vi "micro_Devices.vi"() -> ()   [LabVIEW 2021]
doc: "André Romero - 2023\nandretec@ifsc.usp.br\nIFSC - USP"
uses:
  Controller.ctl
  Thorlabs-Vector-Move/aptTec/Thorlabs-V2/Global Motors.vi
panel:
  out "Z ini":dbl
  out "Array Structures Ind":refnum<vi>[](array[refnum])
  in  "Tab Control":T1(tab)=enum."Cubes"
  in  "start-stop":bool
  in  "step size (mm)":dbl=10.0
  in  "Min   Z":bool
  in  "Max  Z":bool
  in  "Min":bool
  in  "Max":bool
  in  "Z (m/s)":dbl=50.0
  in  "XY (m/s)":dbl format="%#_5g"
  out "Motor Y":bool=TRUE
  out "Motor X":bool=TRUE
  out "Motor Z":bool=TRUE
  in  "Motor - Z":refnum<k7>(container)
  in  "Motor - Y":refnum<k7>(container)
  in  "Motor - X":refnum<k7>(container)
  out "current cube":i32
  out "current Layer":i32=1
  out "Total Progress (%)":u8(slide) caption="Layer Progress (%)" scale=0.0..25.0
  out "Layer Progress (%)":u8(slide)=100 scale=0.0..100.0
  in  "Line step size (mm)":dbl=1.0
  out "Lines Progress (%)":u8(slide)=42 scale=0.0..100.0
  in  "Stop Button":bool
  in  "Go Cubes":bool
  in  "Array of Structures":bool
  in  "Velocity (m/s)":dbl=50.0
  out "Layers":dbl=1.0
  in  "Delta Y (um)":dbl=50.0
  in  "Delta X (um)":dbl=50.0
  in  "Number of Lines":i32=2
  in  "Number of Columns":i32=5
  in  "Layer height (mm)":dbl=1.0
  in  "Height (mm)":dbl=1.0
  in  "Length (mm)":dbl=20.0
  in  "Width (mm)":dbl=20.0
  out "X ini":dbl
  out "Y ini":dbl
  in  "Initial position Z":bool=TRUE
  in  "Z offset (mm)":dbl=10.0
  in  "Z offset":bool
  in  "Motor - Z2":refnum<k7>(container)
  in  "N Loops":i32=5
  in  "Velocity (m/s)":dbl=50.0
  in  "Line step size (mm)":dbl=1.0
  in  "Layer height (mm)":dbl=1.0
  in  "Height (mm)":dbl=5.0
  in  "Length (mm)":dbl=20.0
  in  "Width (mm)":dbl=20.0
  in  "Go Lens":bool
  in  "Release":bool
  out "Numeric":i32
  out "error out":errorcluster
  out "Position Z":sgl
  out "Position Y":dbl
  out "Position X":dbl
  in  "Scale (um)":dbl
  out "XY Graph":cluster{dbl[], dbl[]}(graph)
  in  "Go Test":bool
  in  "Density points":i32
  in  "Velocity (m/s)":dbl=50.0
  in  "círculos":i32
  in  "layers":i32
  in  "scale  z (um)":dbl
  # "Velocity"
  # "Jog"
  # "mm"
  # "Z"
  # "Settings"
  # "Control"
  # "Settings"
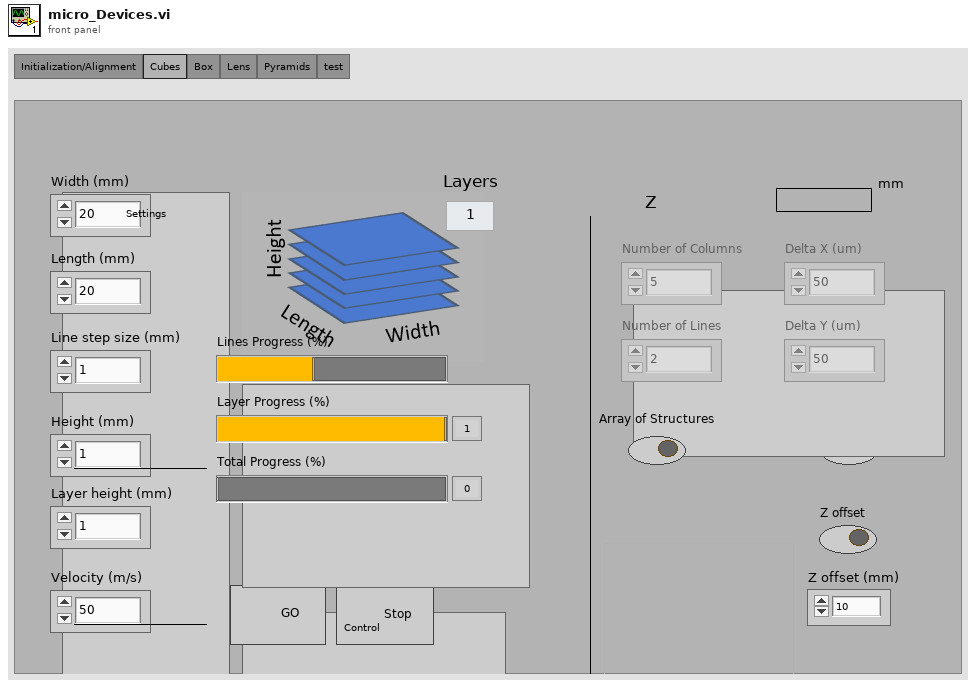
[diagram p1: front panel]
types:
  T1 = enum32{"Initialization/Alignment", "Cubes", "Box", "Lens", "Pyramids", "test"}
  T2 = typedef "Controller.ctl" = enum16{"Initialize", "Wait for Event", "Cubes", "Lens", "Box", "test tap"}
  T3 = typedef "eventvkey.ctl" = enum16{"ASCII", "Enter", "Return", "Shift", "Ctrl", "Alt", "Cmd", "Opt", "Caps", "NumLock", "Clear", "Break", "Up", "Down", "Left", "Right", "Insert", "Delete", "Home", "End", "PageUp", "PageDown", "Escape", "Help", "Pause", "ScrollLock", "F1", "F2", "F3", "F4", "F5", "F6", "F7", "F8", "F9", "F10", "F11", "F12", "F13", "F14", "F15", "F16", "F17", "F18", "F19", "F20", "F21", "F22", "F23", "F24", "Play", "VolumeUp", "VolumeDown", "Mute", "Two Byte Char"}
  T4 = enum8{"Enabled", "Disabled", "Disabled and Grayed Out"}
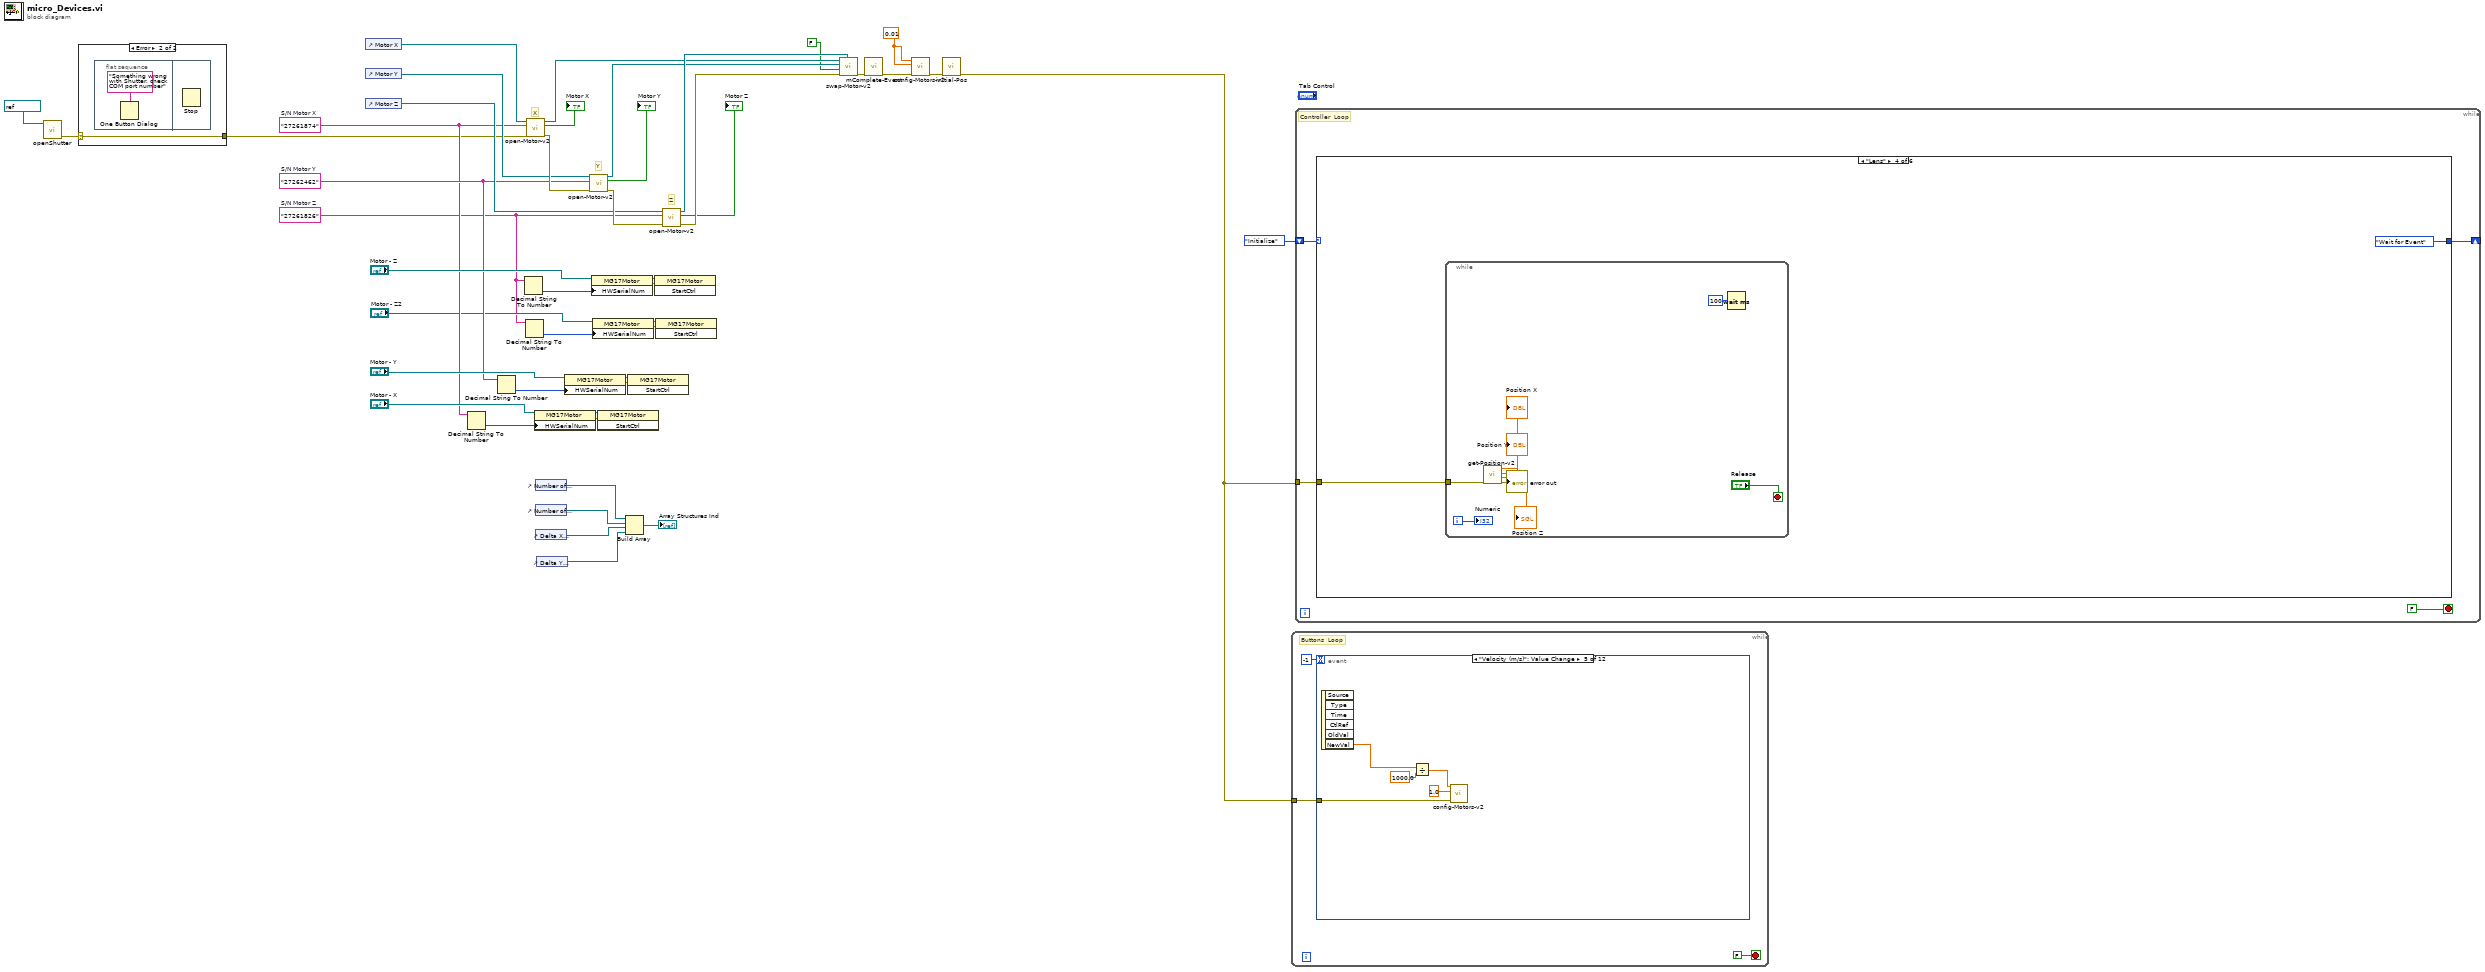
[diagram p0: block diagram]
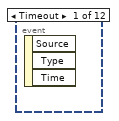
[diagram p3: hidden frame]
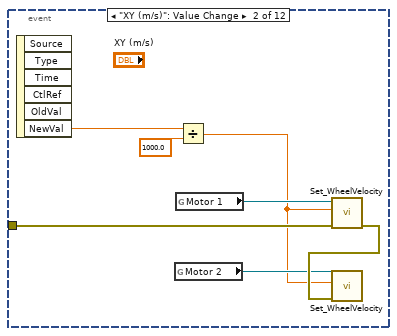
[diagram p4: hidden frame]
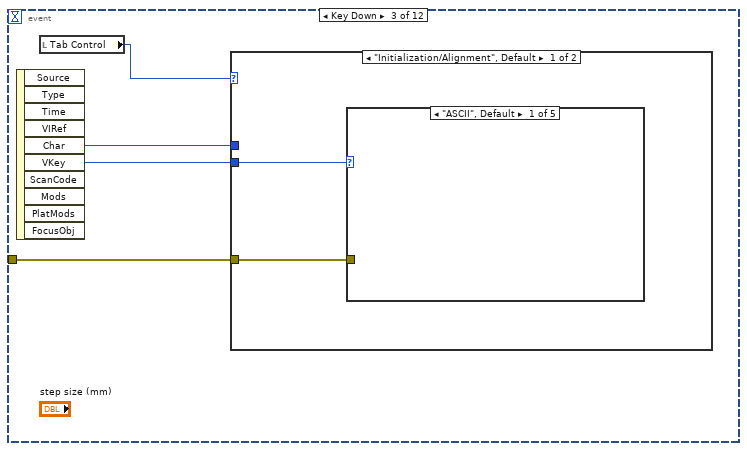
[diagram p5: hidden frame]
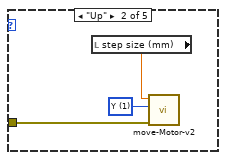
[diagram p6: hidden frame]
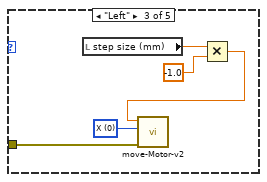
[diagram p7: hidden frame]
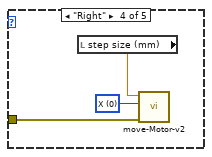
[diagram p8: hidden frame]
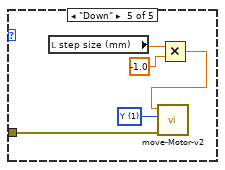
[diagram p9: hidden frame]
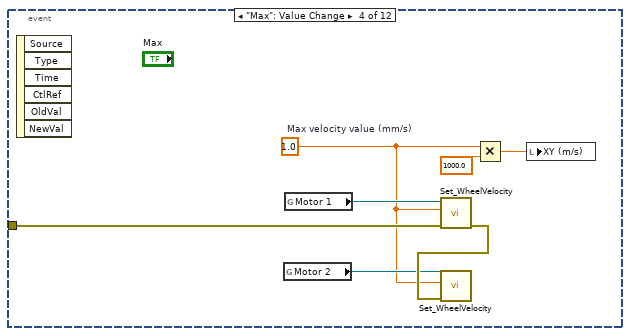
[diagram p11: hidden frame]
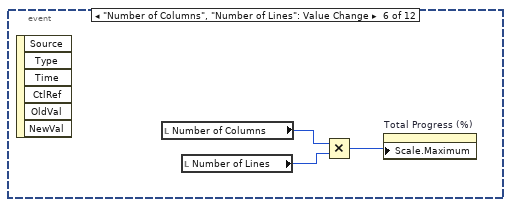
[diagram p12: hidden frame]
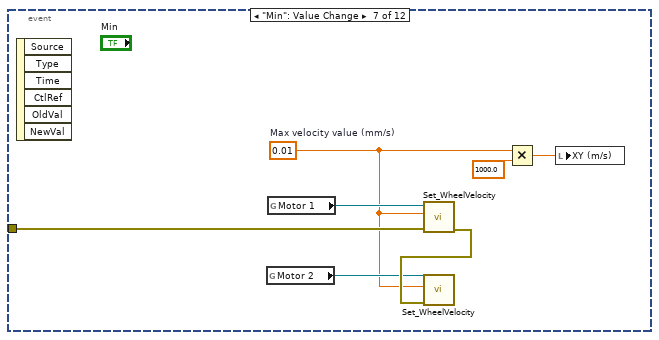
[diagram p13: hidden frame]
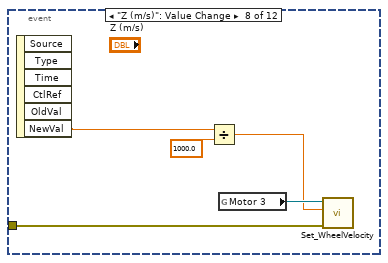
[diagram p14: hidden frame]
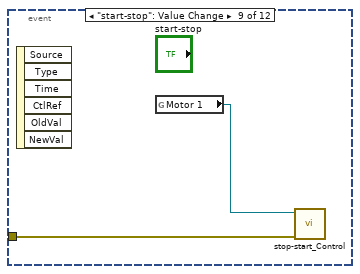
[diagram p15: hidden frame]
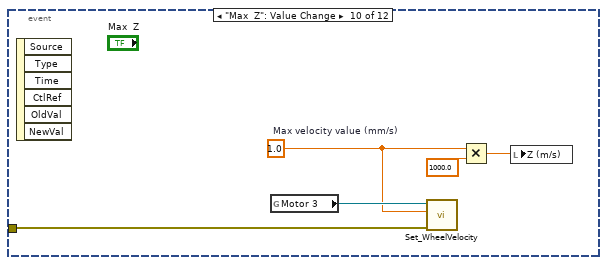
[diagram p16: hidden frame]
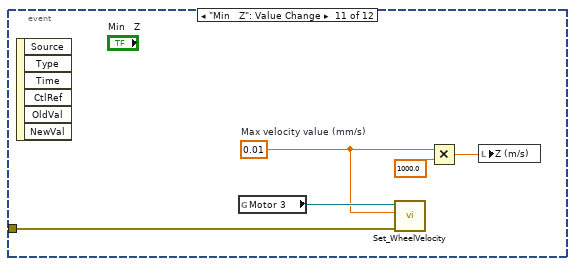
[diagram p17: hidden frame]
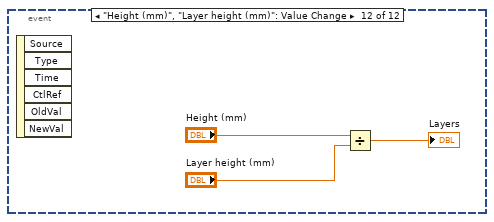
[diagram p18: hidden frame]
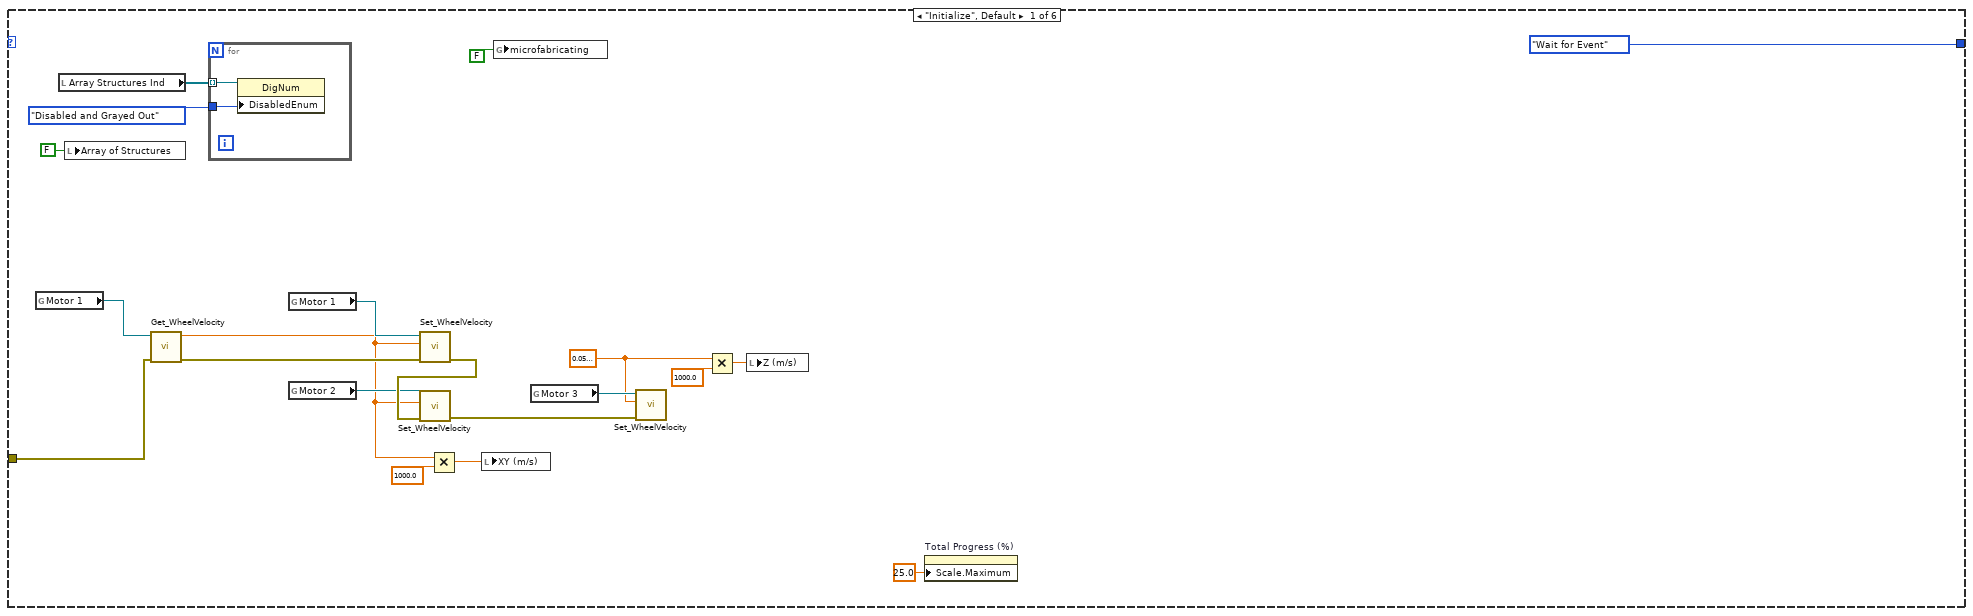
[diagram p19: hidden frame]
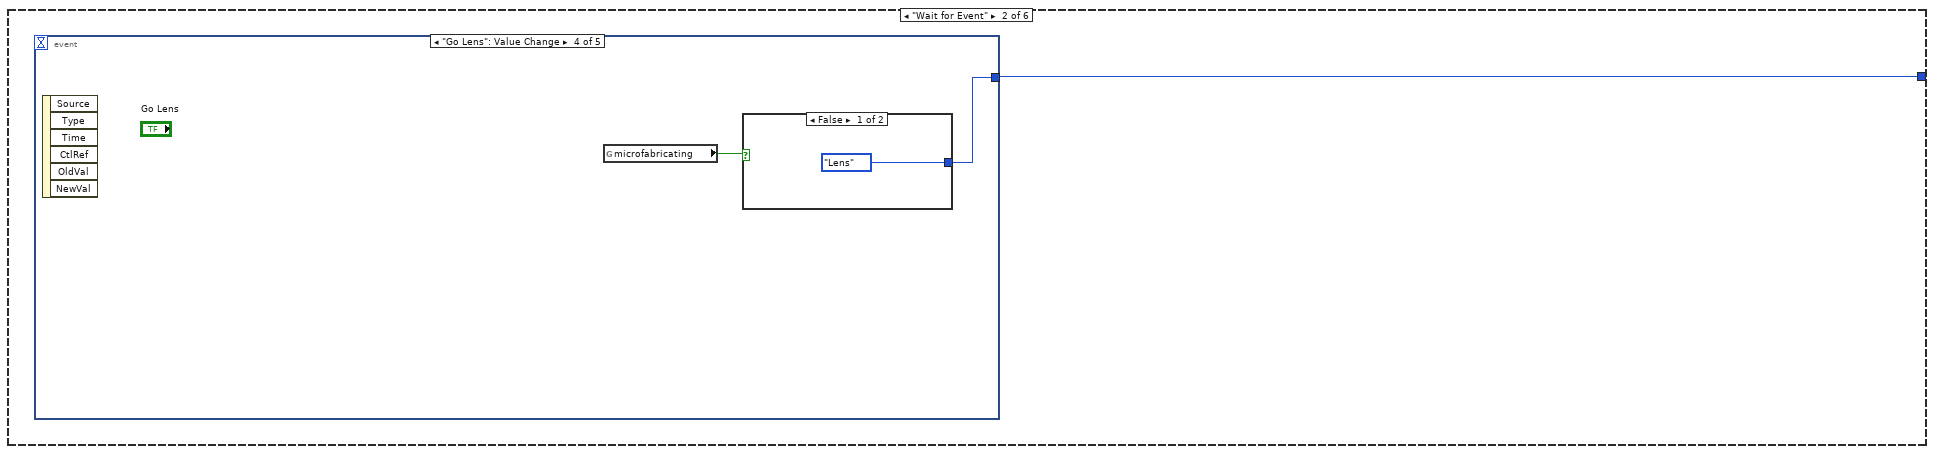
[diagram p20: hidden frame]
diagram:
  w29 = 0.01 ("Acc")
  w16 = "27262462"  # S/N Motor Y
  w15 = "27261874"  # S/N Motor X
  w1 = "27261826"  # S/N Motor Z
  # "X"
  # "Y"
  # "Z"
  n1 = call "openShutter.vi"("VISA Refnum in"=refnum<visa-resource-name> "COM3") -> ("error out"=w7:errorcluster)  [unwired: 9 in, 1 out]
  n2 = case shown="Error" w7 {
    selector: w7 -> [w47 w48]
    tunnel: [w47 w48] -> w6
    frame No Error {
    }
    frame Error {
      n3 = flat-sequence {
        frame #0 {
          n4 = One Button Dialog(message="Something wrong with Shutter, check COM port number") -> ()  [unwired: 1 in, 1 out]
        }
        frame #1 {
          n5 = Stop() -> ()  [unwired: 1 in]
        }
      }
    }
  }
  n6 = control-ref of="Motor X"() -> (w43:refnum<vi>)
  n7 = control-ref of="Motor Y"() -> (w42:refnum<vi>)
  n8 = control-ref of="Motor Z"() -> (w38:refnum<vi>)
  n9 = Decimal String To Number(string=w15) -> (number=w17:i32)  [unwired: 2 in, 1 out]
  n10 = Decimal String To Number(string=w16) -> (number=w21:i32)  [unwired: 2 in, 1 out]
  n11 = Decimal String To Number(string=w1) -> (number=w25:i32)  [unwired: 2 in, 1 out]
  n12 = Decimal String To Number(string=w1) -> (number=w2:i32)  [unwired: 2 in, 1 out]
  n13 = call "open-Motor-v2.vi"("Error In"=w6, "S/N Motor"=w15, "ref Boolean in"=w43) -> ("Error Out"=w46:errorcluster, "Motor Status"=→"Motor X":bool, "Refnum out"=w11:refnum<k7>)  [unwired: 6 in]
  n14 = property class="MG17Motor"(reference="Motor - X", "HWSerialNum"=w17) -> (reference out=w18:refnum<k7>, error out=w19:errorcluster)  [unwired: 1 in]
  n15 = control-ref of="Number of Lines"() -> (w34:refnum<vi>)
  n16 = control-ref of="Number of Columns"() -> (w33:refnum<vi>)
  n17 = control-ref of="Delta X (um)"() -> (w32:refnum<vi>)
  n18 = control-ref of="Delta Y (um)"() -> (w31:refnum<vi>)
  n19 = property class="MG17Motor"(reference="Motor - Y", "HWSerialNum"=w21) -> (reference out=w22:refnum<k7>, error out=w23:errorcluster)  [unwired: 1 in]
  n20 = call "open-Motor-v2.vi"("Error In"=w46, "S/N Motor"=w16, "ref Boolean in"=w42) -> ("Error Out"=w40:errorcluster, "Motor Status"=→"Motor Y":bool, "Refnum out"=w10:refnum<k7>)  [unwired: 6 in]
  n21 = property class="MG17Motor"(reference="Motor - Z", "HWSerialNum"=w25) -> (reference out=w26:refnum<k7>, error out=w27:errorcluster)  [unwired: 1 in]
  n22 = property class="MG17Motor"(reference="Motor - Z2", "HWSerialNum"=w2) -> (reference out=w3:refnum<k7>, error out=w4:errorcluster)  [unwired: 1 in]
  n23 = invoke class="MG17Motor" method="StartCtrl"(reference=w18, error in=w19) -> ()  [unwired: 1 in, 3 out]
  n24 = Build Array(w34, w33, w32, w31) -> (→"Array Structures Ind":refnum<vi>[])
  n25 = invoke class="MG17Motor" method="StartCtrl"(reference=w22, error in=w23) -> ()  [unwired: 1 in, 3 out]
  n26 = invoke class="MG17Motor" method="StartCtrl"(reference=w26, error in=w27) -> ()  [unwired: 1 in, 3 out]
  n27 = invoke class="MG17Motor" method="StartCtrl"(reference=w3, error in=w4) -> ()  [unwired: 1 in, 3 out]
  n28 = call "open-Motor-v2.vi"("Error In"=w40, "S/N Motor"=w1, "ref Boolean in"=w38) -> ("Error Out"=w39:errorcluster, "Motor Status"=→"Motor Z":bool, "Refnum out"=w36:refnum<k7>)  [unwired: 6 in]
  n29 = call "swap-Motor-v2.vi"("Refnum in M3"=w36, "error in (no error)"=w39, "Swap motor"=FALSE, "Refnum in M2"=w10, "Refnum in M1"=w11) -> ("error out"=w14:errorcluster)  [unwired: 6 in]
  n30 = call "mComplete-Event.vi"("Error In"=w14) -> ("Error Out"=w13:errorcluster)  [unwired: 10 in]
  n31 = call "config-Motors-v2.vi"("error in"=w13, "Acc"=w29, "Velocity"=w29) -> ("error out"=w41:errorcluster)  [unwired: 8 in]
  n32 = call "initial-Pos.vi"("error in (no error)"=w41) -> ("error out"=w12:errorcluster)  [unwired: 10 in]
  n33 = while {
    tunnel: w12 -> [w51]
    stop <- FALSE stop-if-true
    # "Buttons  Loop"
    n34 = event shown="[4] \"Velocity (m/s)\": Value Change" {
      selector: _ -> [_ _ _ _ _ _ _ _ _ _ _ _]
      dyn-events: _ -> [_ _ _ _ _ _ _ _ _ _ _ _]
      timeout: -1 -> [_ _ _ _ _ _ _ _ _ _ _ _]
      tunnel: w51 -> [_ w58 w60 w85 w89 _ w100 w104 w110 w111 w116 _]
      event Timeout {
        n35 = event-data() -> ()  [unwired: 1 in, 3 out]
      }
      event "XY (m/s)": Value Change {
        n36 = event-data() -> ("NewVal"=w55:dbl)  [unwired: 1 in, 5 out]
        n37 = global read "Global Motors.vi" "Motor 2"() -> (w56:refnum<k7>)
        n38 = global read "Global Motors.vi" "Motor 1"() -> (w59:refnum<k7>)
        n39 = Divide(x=w55, y=1000.0) -> (x/y=w54:dbl)
        n40 = call "Set_WheelVelocity.vi"("error in"=w58, "fWheelVel"=w54, "MG17Motor in"=w59) -> ("error out"=w57:errorcluster)  [unwired: 8 in]
        n41 = call "Set_WheelVelocity.vi"("error in"=w57, "fWheelVel"=w54, "MG17Motor in"=w56) -> ()  [unwired: 8 in, 1 out]
      }
      event Key Down {
        n42 = event-data() -> ("Char"=w62:i16, "VKey"=w61:T3)  [unwired: 1 in, 8 out]
        n43 = local read "Tab Control"() -> (w63:T1)
        n44 = case shown="\"Initialization/Alignment\", Default" w63 {
          tunnel: w62 -> [_ _]
          tunnel: w61 -> [w65 _]
          tunnel: w60 -> [w64 _]
          frame "Initialization/Alignment", Default {
            n45 = case shown="\"ASCII\", Default" w65 {
              tunnel: w64 -> [_ w68 w73 w76 w80]
              frame "ASCII", Default {
              }
              frame "Up" {
                w67 = u16 1 items=["X", "Y", "Z"] ("Axis")
                n46 = local read "step size (mm)"() -> (w66:dbl)
                n47 = call "move-Motor-v2.vi"("error in"=w68, "Axis"=w67, "Distance (um)"=w66) -> ()  [unwired: 8 in, 1 out]
              }
              frame "Left" {
                w72 = u16 0 items=["X", "Y", "Z"] ("Axis")
                n48 = local read "step size (mm)"() -> (w71:dbl)
                n49 = Multiply(x=w71, y=-1.0) -> (x*y=w69:dbl)
                n50 = call "move-Motor-v2.vi"("error in"=w73, "Axis"=w72, "Distance (um)"=w69) -> ()  [unwired: 8 in, 1 out]
              }
              frame "Right" {
                w75 = u16 0 items=["X", "Y", "Z"] ("Axis")
                n51 = local read "step size (mm)"() -> (w74:dbl)
                n52 = call "move-Motor-v2.vi"("error in"=w76, "Axis"=w75, "Distance (um)"=w74) -> ()  [unwired: 8 in, 1 out]
              }
              frame "Down" {
                w81 = u16 1 items=["X", "Y", "Z"] ("Axis")
                n53 = local read "step size (mm)"() -> (w79:dbl)
                n54 = Multiply(x=w79, y=-1.0) -> (x*y=w77:dbl)
                n55 = call "move-Motor-v2.vi"("error in"=w80, "Axis"=w81, "Distance (um)"=w77) -> ()  [unwired: 8 in, 1 out]
              }
            }
          }
          frame "Cubes" {
          }
        }
      }
      event "Max": Value Change {
        w83 = 1.0  # Max velocity value (mm/s)
        n56 = event-data() -> ()  [unwired: 1 in, 6 out]
        n57 = global read "Global Motors.vi" "Motor 2"() -> (w86:refnum<k7>)
        n58 = global read "Global Motors.vi" "Motor 1"() -> (w88:refnum<k7>)
        n59 = call "Set_WheelVelocity.vi"("error in"=w85, "fWheelVel"=w83, "MG17Motor in"=w88) -> ("error out"=w87:errorcluster)  [unwired: 8 in]
        n60 = call "Set_WheelVelocity.vi"("error in"=w87, "fWheelVel"=w83, "MG17Motor in"=w86) -> ()  [unwired: 8 in, 1 out]
        n61 = Multiply(x=w83, y=1000.0) -> (x*y=w82:dbl)
        n62 = local write "XY (m/s)"(w82) -> ()
      }
      event "Velocity (m/s)": Value Change {
        n63 = event-data() -> ("NewVal"=w93:dbl)  [unwired: 1 in, 5 out]
        n64 = Divide(x=w93, y=1000.0) -> (x/y=w91:dbl)
        n65 = call "config-Motors-v2.vi"("error in"=w89, "Acc"=1.0, "Velocity"=w91) -> ()  [unwired: 8 in, 1 out]
      }
      event "Number of Columns", "Number of Lines": Value Change {
        n66 = event-data() -> ()  [unwired: 1 in, 6 out]
        n67 = local read "Number of Columns"() -> (w95:i32)
        n68 = local read "Number of Lines"() -> (w96:i32)
        n69 = Multiply(x=w95, y=w96) -> (x*y=w94:i32)
        n70 = property on="Total Progress (%)" class="Slide (strict)"("Scale.Maximum"=w94) -> ()  [unwired: 2 in, 2 out]
      }
      event "Min": Value Change {
        w98 = 0.01  # Max velocity value (mm/s)
        n71 = event-data() -> ()  [unwired: 1 in, 6 out]
        n72 = global read "Global Motors.vi" "Motor 2"() -> (w101:refnum<k7>)
        n73 = global read "Global Motors.vi" "Motor 1"() -> (w103:refnum<k7>)
        n74 = call "Set_WheelVelocity.vi"("error in"=w100, "fWheelVel"=w98, "MG17Motor in"=w103) -> ("error out"=w102:errorcluster)  [unwired: 8 in]
        n75 = call "Set_WheelVelocity.vi"("error in"=w102, "fWheelVel"=w98, "MG17Motor in"=w101) -> ()  [unwired: 8 in, 1 out]
        n76 = Multiply(x=w98, y=1000.0) -> (x*y=w97:dbl)
        n77 = local write "XY (m/s)"(w97) -> ()
      }
      event "Z (m/s)": Value Change {
        n78 = event-data() -> ("NewVal"=w107:dbl)  [unwired: 1 in, 5 out]
        n79 = Divide(x=w107, y=1000.0) -> (x/y=w105:dbl)
        n80 = global read "Global Motors.vi" "Motor 3"() -> (w106:refnum<k7>)
        n81 = call "Set_WheelVelocity.vi"("error in"=w104, "fWheelVel"=w105, "MG17Motor in"=w106) -> ()  [unwired: 8 in, 1 out]
      }
      event "start-stop": Value Change {
        n82 = event-data() -> ()  [unwired: 1 in, 6 out]
        n83 = global read "Global Motors.vi" "Motor 1"() -> (w109:refnum<k7>)
        n84 = call "stop-start_Control.vi"("error in (no error)"=w110, "Automation Refnum in"=w109) -> ()  [unwired: 8 in, 2 out]
      }
      event "Max  Z": Value Change {
        w113 = 1.0  # Max velocity value (mm/s)
        n85 = event-data() -> ()  [unwired: 1 in, 6 out]
        n86 = global read "Global Motors.vi" "Motor 3"() -> (w115:refnum<k7>)
        n87 = call "Set_WheelVelocity.vi"("error in"=w111, "fWheelVel"=w113, "MG17Motor in"=w115) -> ()  [unwired: 8 in, 1 out]
        n88 = Multiply(x=w113, y=1000.0) -> (x*y=w112:dbl)
        n89 = local write "Z (m/s)"(w112) -> ()
      }
      event "Min   Z": Value Change {
        w118 = 0.01  # Max velocity value (mm/s)
        n90 = event-data() -> ()  [unwired: 1 in, 6 out]
        n91 = global read "Global Motors.vi" "Motor 3"() -> (w120:refnum<k7>)
        n92 = call "Set_WheelVelocity.vi"("error in"=w116, "fWheelVel"=w118, "MG17Motor in"=w120) -> ()  [unwired: 8 in, 1 out]
        n93 = Multiply(x=w118, y=1000.0) -> (x*y=w117:dbl)
        n94 = local write "Z (m/s)"(w117) -> ()
      }
      event "Height (mm)", "Layer height (mm)": Value Change {
        n95 = event-data() -> ()  [unwired: 1 in, 6 out]
        n96 = Divide(x="Height (mm)", y="Layer height (mm)") -> (x/y=→"Layers":dbl)
      }
    }
  }
  n97 = while {
    shift-right: [w125] -> _
    shift-left: Controller."Initialize" -> [w126]
    tunnel: w12 -> [w124]
    stop <- FALSE stop-if-true
    # "Controller  Loop"
    n98 = case shown="\"Lens\"" w126 {
      tunnel: [Controller."Wait for Event" w150 Controller."Wait for Event" Controller."Wait for Event" Controller."Wait for Event" w362] -> w125
      tunnel: w124 -> [w129 _ w191 w326 w338 w355]
      frame "Initialize", Default {
        w133 = sgl 0.05 ("fWheelVel")
        n99 = global read "Global Motors.vi" "Motor 1"() -> (w143:refnum<k7>)
        n100 = local read "Array Structures Ind"() -> (w145:refnum<vi>[])
        n101 = local write "Array of Structures"(FALSE ("Array of Structures")) -> ()
        n102 = call "Get_WheelVelocity.vi"("error in"=w129, "MG17Motor in"=w143) -> ("error out"=w139:errorcluster, "pfWheelVel"=w138:sgl)  [unwired: 8 in]
        n103 = for {
          tunnel: T4."Disabled and Grayed Out" ("Disabled") -> [w149]
          tunnel: w145 -> [w148] mode=indexing
          n104 = property class="DigNum"(reference=w148, "DisabledEnum"=w149) -> ()  [unwired: 1 in, 2 out]
        }
        n105 = global read "Global Motors.vi" "Motor 1"() -> (w142:refnum<k7>)
        n106 = global read "Global Motors.vi" "Motor 2"() -> (w140:refnum<k7>)
        n107 = call "Set_WheelVelocity.vi"("error in"=w139, "fWheelVel"=w138, "MG17Motor in"=w142) -> ("error out"=w141:errorcluster)  [unwired: 8 in]
        n108 = call "Set_WheelVelocity.vi"("error in"=w141, "fWheelVel"=w138, "MG17Motor in"=w140) -> ("error out"=w135:errorcluster)  [unwired: 8 in]
        n109 = Multiply(x=w138, y=sgl 1000.0) -> (x*y=w137:sgl)
        n110 = local write "XY (m/s)"(w137) -> ()
        n111 = global write "Global micro_Devices.vi" "microfabricating"(FALSE ("microfabricating")) -> ()
        n112 = global read "Global Motors.vi" "Motor 3"() -> (w134:refnum<k7>)
        n113 = call "Set_WheelVelocity.vi"("error in"=w135, "fWheelVel"=w133, "MG17Motor in"=w134) -> ()  [unwired: 8 in, 1 out]
        n114 = Multiply(x=w133, y=sgl 1000.0) -> (x*y=w132:sgl)
        n115 = local write "Z (m/s)"(w132) -> ()
        n116 = property on="Total Progress (%)" class="Slide (strict)"("Scale.Maximum"=25.0 ("Scale.Range:Maximum")) -> ()  [unwired: 2 in, 2 out]
      }
      frame "Wait for Event" {
        n117 = event shown="[3] \"Go Lens\": Value Change" {
          selector: _ -> [_ _ _ _ _]
          dyn-events: _ -> [_ _ _ _ _]
          timeout: _ -> [_ _ _ _ _]
          tunnel: [Controller."Wait for Event" Controller."Wait for Event" w160 w164 w168] -> w150
          event Timeout {
            n118 = event-data() -> ()  [unwired: 1 in, 3 out]
          }
          event "Array of Structures": Value Change {
            n119 = event-data() -> ("NewVal"=w153:bool)  [unwired: 1 in, 5 out]
            n120 = case shown="False" w153 {
              tunnel: [T4."Disabled and Grayed Out" ("Disabled") T4."Enabled" ("Disabled")] -> w154
              frame False {
              }
              frame True {
              }
            }
            n121 = local read "Array Structures Ind"() -> (w155:refnum<vi>[])
            n122 = for {
              tunnel: w154 -> [w157]
              tunnel: w155 -> [w156] mode=indexing
              n123 = property class="DigNum"(reference=w156, "DisabledEnum"=w157) -> ()  [unwired: 1 in, 2 out]
            }
          }
          event "Go Cubes": Value Change {
            n124 = event-data() -> ()  [unwired: 1 in, 6 out]
            n125 = global read "Global micro_Devices.vi" "microfabricating"() -> (w161:bool)
            n126 = case shown="False" w161 {
              tunnel: [Controller."Cubes" Controller."Wait for Event"] -> w160
              frame False {
              }
              frame True {
              }
            }
          }
          event "Go Lens": Value Change {
            n127 = event-data() -> ()  [unwired: 1 in, 6 out]
            n128 = global read "Global micro_Devices.vi" "microfabricating"() -> (w165:bool)
            n129 = case shown="False" w165 {
              tunnel: [Controller."Lens" Controller."Wait for Event"] -> w164
              frame False {
              }
              frame True {
              }
            }
          }
          event "Go Test": Value Change {
            n130 = event-data() -> ()  [unwired: 1 in, 6 out]
            n131 = global read "Global micro_Devices.vi" "microfabricating"() -> (w169:bool)
            n132 = case shown="True" w169 {
              tunnel: [Controller."test tap" Controller."Wait for Event"] -> w168
              frame False {
              }
              frame True {
              }
            }
          }
        }
      }
      frame "Cubes" {
        w178 = u16 1 items=["X", "Y", "Z"] ("Axis")
        w177 = 0.0 ("Distance (um)")
        w180 = u16 0 items=["X", "Y", "Z"] ("Axis")
        # "Initial Settings"
        # "Backlash"
        n133 = global write "Global micro_Devices.vi" "Current Cube"(1 ("Current Cube")) -> ()
        n134 = global write "Global micro_Devices.vi" "microfabricating"(FALSE ("microfabricating")) -> ()
        n135 = Divide(x="Velocity (m/s)", y=1000.0) -> (x/y=w182:dbl)
        n136 = call "config-Motors-v2.vi"("error in"=w191, "Acc"=1.0, "Velocity"=w182) -> ("error out"=w176:errorcluster)  [unwired: 8 in]
        n137 = call "move-Motor-v2.vi"("error in"=w176, "Axis"=w180, "Distance (um)"=w177) -> ("error out"=w179:errorcluster)  [unwired: 8 in]
        n138 = call "move-Motor-v2.vi"("error in"=w179, "Axis"=w178, "Distance (um)"=w177) -> ("error out"=w175:errorcluster)  [unwired: 8 in]
        n139 = Multiply(x=1.0, y="Width (mm)") -> (x*y=w173:dbl)
        n140 = local read "Array of Structures"() -> (w186:bool)
        n141 = call "initial-Pos-XY.vi"("error in (no error)"=w175) -> ("error out"=w188:errorcluster, "Y position"=w184:dbl, "X position"=w185:dbl)  [unwired: 8 in]
        n142 = Divide(x="Length (mm)", y="Line step size (mm)") -> (x/y=w193:dbl)
        n143 = call "initial-Pos-Z.vi"("error in (no error)"=w188) -> ("error out"=w187:errorcluster, "Z position"=w183:dbl)  [unwired: 9 in]
        n144 = case shown="True" w186 {
          tunnel: w173 -> [w203 w238]
          tunnel: w193 -> [w202 w239]
          tunnel: "Line step size (mm)" -> [w201 w237]
          tunnel: w187 -> [w200 w236]
          tunnel: w185 -> [_ w235]
          tunnel: w184 -> [_ w234]
          tunnel: w183 -> [_ w233]
          frame False {
            n145 = while {
              tunnel: w203 -> [w225]
              tunnel: w202 -> [w224]
              tunnel: w201 -> [w223]
              tunnel: w200 -> [w221]
              tunnel: [w214] -> w199
              i -> [w217]
              stop <- w216 stop-if-true
              n146 = call "toggleShutter.vi"("Error In"=w221) -> ("error out"=w220:errorcluster)  [unwired: 9 in]
              n147 = Increment(x=w217) -> (x+1=w212:i32)
              "current Layer" <- w212
              n148 = local read "Layer height (mm)"() -> (w208:dbl)
              n149 = local read "Height (mm)"() -> (w207:dbl)
              n150 = control-ref of="Lines Progress (%)"() -> (w222:refnum<vi>)
              n151 = Multiply(x=100.0, y=w212) -> (x*y=w211:dbl)
              n152 = call "make-Lines.vi"("Shutter off between lines"=TRUE, "Slide in"=w222, "error in"=w220, "d (um)"=w223, "L (um)"=w225, "N Lines"=w224) -> ("error out"=w219:errorcluster)  [unwired: 4 in, 1 out]
              n153 = call "toggleShutter.vi"("Error In"=w219) -> ("error out"=w218:errorcluster)  [unwired: 9 in]
              n154 = local read "Layers"() -> (w210:dbl)
              n155 = Equal?(x=w207, y=w208) -> (x = y?=w206:bool)
              n156 = Divide(x=w211, y=w210) -> (x/y=→"Layer Progress (%)":dbl)
              n157 = case shown="False" w206 {
                tunnel: w218 -> [w228 w230]
                tunnel: [w227 w230] -> w215
                tunnel: w208 -> [w226 _]
                frame False {
                  w229 = u16 2 items=["X", "Y", "Z"] ("Axis")
                  n158 = call "move-Motor-v2.vi"("error in"=w228, "Axis"=w229, "Distance (um)"=w226) -> ("error out"=w227:errorcluster)  [unwired: 8 in]
                }
                frame True {
                }
              }
              n159 = Equal?(x=w210, y=w212) -> (x = y?=w216:bool)
              n160 = call "moveXYToInitialPos.vi"("error in"=w215) -> ("error out"=w214:errorcluster)  [unwired: 10 in]
            }
            n161 = case shown="True" "Initial position Z" {
              tunnel: w199 -> [_ w204]
              frame False {
              }
              frame True {
                n162 = call "moveZToInitialPos.vi"("error in"=w204) -> ()  [unwired: 10 in, 1 out]
              }
            }
          }
          frame True {
            n163 = while {
              tunnel: w239 -> [w260]
              tunnel: w238 -> [w259]
              tunnel: w237 -> [w258]
              tunnel: w236 -> [w257]
              tunnel: [w241] -> w231
              i -> [w254]
              stop <- w253 stop-if-true
              w252 = u16 1 items=["X", "Y", "Z"] ("Axis")
              n164 = while {
                tunnel: w260 -> [w289]
                tunnel: w259 -> [w288]
                tunnel: w258 -> [w287]
                tunnel: w257 -> [w286]
                tunnel: [w269] -> w242
                i -> [w279]
                stop <- w277 stop-if-true
                w284 = u16 0 items=["X", "Y", "Z"] ("Axis")
                n165 = global read "Global micro_Devices.vi" "Current Cube"() -> (w261:i32)
                "current cube" <- w261
                "Total Progress (%)" <- w261
                n166 = while {
                  tunnel: w289 -> [w317]
                  tunnel: w288 -> [w316]
                  tunnel: w287 -> [w315]
                  tunnel: w286 -> [w314]
                  tunnel: [w312] -> w285
                  i -> [w307]
                  stop <- w306 stop-if-true
                  n167 = control-ref of="Lines Progress (%)"() -> (w305:refnum<vi>)
                  n168 = call "toggleShutter.vi"("Error In"=w314) -> ("error out"=w313:errorcluster)  [unwired: 9 in]
                  n169 = Increment(x=w307) -> (x+1=w304:i32)
                  n170 = local read "Layer height (mm)"() -> (w302:dbl)
                  n171 = local read "Height (mm)"() -> (w301:dbl)
                  n172 = call "make-Lines.vi"("Shutter off between lines"=TRUE, "Slide in"=w305, "error in"=w313, "d (um)"=w315, "L (um)"=w316, "N Lines"=w317) -> ("error out"=w320:errorcluster)  [unwired: 4 in, 1 out]
                  n173 = Multiply(x=100.0, y=w304) -> (x*y=w309:dbl)
                  n174 = call "toggleShutter.vi"("Error In"=w320) -> ("error out"=w319:errorcluster)  [unwired: 9 in]
                  n175 = local write "current Layer"(w304) -> ()
                  n176 = Equal?(x=w302, y=w301) -> (x = y?=w303:bool)
                  n177 = local read "Layers"() -> (w310:dbl)
                  n178 = case shown="False" w303 {
                    tunnel: w319 -> [w323 w325]
                    tunnel: [w322 w325] -> w318
                    tunnel: w302 -> [w321 _]
                    frame False {
                      w324 = u16 2 items=["X", "Y", "Z"] ("Axis")
                      n179 = call "move-Motor-v2.vi"("error in"=w323, "Axis"=w324, "Distance (um)"=w321) -> ("error out"=w322:errorcluster)  [unwired: 8 in]
                    }
                    frame True {
                    }
                  }
                  n180 = Divide(x=w309, y=w310) -> (x/y=w308:dbl)
                  n181 = local write "Layer Progress (%)"(w308) -> ()
                  n182 = Greater Or Equal?(x=w310, y=w304) -> (x >= y?=w306:bool)
                  n183 = call "moveXYToInitialPos.vi"("error in"=w318) -> ("error out"=w312:errorcluster)  [unwired: 10 in]
                }
                n184 = Increment(x=w261) -> (x+1=w274:i32)
                n185 = global write "Global micro_Devices.vi" "Current Cube"(w274) -> ()
                n186 = local read "Width (mm)"() -> (w282:dbl)
                n187 = Multiply(x="Delta X (um)", y=1.0) -> (x*y=w273:dbl)
                n188 = Add(x=w282, y=w273) -> (x+y=w280:dbl)
                n189 = call "moveZToInitialPos.vi"("error in"=w285) -> ("error out"=w283:errorcluster)  [unwired: 10 in]
                n190 = global read "Global micro_Devices.vi" "Current Cube"() -> (w266:i32)
                n191 = local read "Z ini"() -> (w265:dbl)
                n192 = call "move-Motor-v2.vi"("error in"=w283, "Axis"=w284, "Distance (um)"=w280) -> ("error out"=w276:errorcluster)  [unwired: 8 in]
                n193 = call "initial-Pos-XY.vi"("error in (no error)"=w276) -> ("error out"=w270:errorcluster)  [unwired: 8 in, 2 out]
                n194 = Increment(x=w279) -> (x+1=w278:i32)
                n195 = Decrement(x=w266) -> (x-1=w267:i32)
                n196 = Multiply(x=w267, y="Z offset (mm)") -> (x*y=w264:dbl)
                n197 = Add(x=w264, y=w265) -> (x+y=w262:dbl)
                n198 = Equal?(x="Number of Columns", y=w278) -> (x = y?=w277:bool)
                n199 = Not Equal To 0?(x=w264) -> (x != 0?=w263:bool)
                n200 = case shown="True" "Z offset" {
                  tunnel: w270 -> [w290 w294]
                  tunnel: [w290 w293] -> w269
                  tunnel: w263 -> [_ w292]
                  tunnel: w262 -> [_ w291]
                  frame False {
                  }
                  frame True {
                    n201 = case shown="True" w292 {
                      tunnel: w294 -> [w295 w298]
                      tunnel: [w295 w297] -> w293
                      tunnel: w291 -> [_ w296]
                      frame False {
                      }
                      frame True {
                        w299 = u16 2 items=["X", "Y", "Z"] ("Axis")
                        n202 = call "move-Motor-v2.vi"("error in"=w298, "Axis"=w299, "Distance (um)"=w296) -> ("error out"=w297:errorcluster)  [unwired: 8 in]
                      }
                    }
                  }
                }
              }
              n203 = Increment(x=w254) -> (x+1=w248:i32)
              n204 = local read "X ini"() -> (w244:dbl)
              n205 = local read "Length (mm)"() -> (w255:dbl)
              n206 = Subtract(x=w244, y=0.02 ("x")) -> (x-y=w247:dbl)
              n207 = call "goToabsX.vi"("error in"=w242, "X position"=w247) -> ("error out"=w245:errorcluster)  [unwired: 9 in]
              n208 = Add(x="Delta Y (um)", y=w255) -> (x+y=w251:dbl)
              n209 = Equal?(x="Number of Lines", y=w248) -> (x = y?=w253:bool)
              n210 = call "goToabsX.vi"("error in"=w245, "X position"=w244) -> ("error out"=w243:errorcluster)  [unwired: 9 in]
              n211 = call "move-Motor-v2.vi"("error in"=w243, "Axis"=w252, "Distance (um)"=w251) -> ("error out"=w250:errorcluster)  [unwired: 8 in]
              n212 = call "initial-Pos-XY.vi"("error in (no error)"=w250) -> ("error out"=w241:errorcluster)  [unwired: 8 in, 2 out]
            }
            n213 = local read "Initial position Z"() -> (w232:bool)
            n214 = case shown="True" w232 {
              tunnel: w231 -> [_ w240]
              frame False {
              }
              frame True {
                n215 = call "moveZToInitialPos.vi"("error in"=w240) -> ()  [unwired: 10 in, 1 out]
              }
            }
            "X ini" <- w235
            "Y ini" <- w234
            "Z ini" <- w233
          }
        }
      }
      frame "Lens" {
        n216 = while {
          tunnel: w326 -> [w332]
          i -> [w334]
          stop <- "Release" stop-if-true
          n217 = call "get-Position-v2.vi"("error in (no error)"=w332) -> ("error out"=→"error out":errorcluster, "Position Z"=→"Position Z":sgl, "Position Y"=→"Position Y":dbl, "Position X"=→"Position X":dbl)  [unwired: 7 in]
          n218 = Wait (ms)(milliseconds to wait=u32 100) -> ()  [unwired: 1 out]
          "Numeric" <- w334
        }
      }
      frame "Box" {
        w342 = u16 1 items=["X", "Y", "Z"] ("Axis")
        w341 = 0.0 ("Distance (um)")
        w344 = u16 0 items=["X", "Y", "Z"] ("Axis")
        # "Backlash"
        n219 = Divide(x="Velocity (m/s)", y=1000.0) -> (x/y=w346:dbl)
        n220 = call "config-Motors-v2.vi"("error in"=w338, "Acc"=1.0, "Velocity"=w346) -> ("error out"=w340:errorcluster)  [unwired: 8 in]
        n221 = call "move-Motor-v2.vi"("error in"=w340, "Axis"=w344, "Distance (um)"=w341) -> ("error out"=w343:errorcluster)  [unwired: 8 in]
        n222 = call "move-Motor-v2.vi"("error in"=w343, "Axis"=w342, "Distance (um)"=w341) -> ("error out"=w339:errorcluster)  [unwired: 8 in]
        n223 = call "initial-Pos-XY.vi"("error in (no error)"=w339) -> ("error out"=w347:errorcluster)  [unwired: 8 in, 2 out]
        n224 = call "initial-Pos-Z.vi"("error in (no error)"=w347) -> ()  [unwired: 9 in, 2 out]
        n225 = for {
          N: "N Loops" -> [_]
        }
      }
      frame "test tap" {
        n226 = Divide(x="Velocity (m/s)", y=1000.0) -> (x/y=w357:dbl)
        n227 = call "config-Motors-v2.vi"("error in"=w355, "Acc"=1.0, "Velocity"=w357) -> ("error out"=w354:errorcluster)  [unwired: 8 in]
        n228 = disable-structure shown="Disabled" {
          disable-tunnel: w354 -> [w411 w416]
          disable-tunnel: [w412 w416] -> w360
          frame Disabled {
            w414 = u16 1 items=["X", "Y", "Z"] ("Axis")
            w415 = u16 0 items=["X", "Y", "Z"] ("Axis")
            w413 = 7.0 ("Distance (um)")
            n229 = call "move-Motor-v2.vi"("error in"=w411, "Axis"=w414, "Distance (um)"=w413) -> ()  [unwired: 8 in, 1 out]
            n230 = call "move-Motor-v2.vi"("error in"=w411, "Axis"=w415, "Distance (um)"=w413) -> ("error out"=w412:errorcluster)  [unwired: 8 in]
          }
          frame Enabled {
          }
        }
        n231 = for {
          N: "Density points" -> [w429]
          tunnel: [w418] -> w353
          tunnel: [w417] -> w352
          tunnel: w360 -> [w421]
          tunnel: [w421] -> w351
          i -> [w427]
          w419 = dbl[] []
          n232 = Divide(x=6.283185307179586, y=w429) -> (x/y=w428:dbl)
          n233 = Multiply(x=w428, y=w427) -> (x*y=w426:dbl)
          n234 = Sine & Cosine(0:w426) -> (1:w420:dbl, 2:w422:dbl)
          n235 = feedback #1(w419) -> (w425:dbl[])
          n236 = Build Array (concatenate)(w425, w420) -> (w418:dbl[])
          n237 = feedback-in #1(w418) -> ()
          n238 = feedback #2(w419) -> (w424:dbl[])
          n239 = Build Array (concatenate)(w424, w422) -> (w417:dbl[])
          n240 = feedback-in #2(w417) -> ()
          n241 = Bundle(w418, w417) -> (→"XY Graph":cluster{dbl[], dbl[]})  [unwired: 1 in]
        }
        n242 = for {
          N: "layers" -> [_]
          tunnel: [Controller."Wait for Event"] -> w362
          tunnel: "Density points" -> [w370]
          tunnel: w353 -> [w369]
          tunnel: w352 -> [w368]
          tunnel: w351 -> [w364]
          w365 = u16 2 items=["X", "Y", "Z"] ("Axis")
          n243 = for {
            N: "círculos" -> [_]
            tunnel: w370 -> [w374]
            tunnel: w369 -> [w390]
            tunnel: w368 -> [w388]
            tunnel: [w372] -> _
            tunnel: [w373] -> w366
            tunnel: w364 -> [w372]
            i -> [w376]
            w385 = u16 1 items=["X", "Y", "Z"] ("Axis")
            w391 = u16 1 items=["X", "Y", "Z"] ("Axis")
            n244 = Increment(x=w376) -> (x+1=w375:i32)
            n245 = Multiply(x="Scale (um)", y=w375) -> (x*y=w386:dbl)
            n246 = Multiply(x=w386, y=w388) -> (x*y=w387:dbl[])
            n247 = Multiply(x=w386, y=w390) -> (x*y=w389:dbl[])
            n248 = Index Array(array=w387, index=0) -> (element=w384:dbl)
            n249 = call "move-Motor-v2.vi"("error in"=w372, "Axis"=w391, "Distance (um)"=w384) -> ("error out"=w381:errorcluster)  [unwired: 8 in]
            n250 = call "toggleShutter.vi"("Error In"=w381) -> ("error out"=w380:errorcluster)  [unwired: 9 in]
            n251 = for {
              N: w374 -> [_]
              tunnel: w387 -> [w410]
              tunnel: w389 -> [w395]
              tunnel: w380 -> [w394]
              tunnel: [w393] -> w379
              i -> [w396]
              w399 = u16 0 items=["X", "Y", "Z"] ("Axis")
              w405 = u16 1 items=["X", "Y", "Z"] ("Axis")
              n252 = Add(x=1 ("x-y"), y=w396) -> (x+y=w402:i32)
              n253 = Add(x=1 ("x-y"), y=w396) -> (x+y=w408:i32)
              n254 = Index Array(array=w395, index #1=w402, index #2=w396) -> (element #1=w401:dbl, element #2=w400:dbl)
              n255 = Index Array(array=w410, index #1=w408, index #2=w396) -> (element #1=w407:dbl, element #2=w406:dbl)
              n256 = Subtract(x=w401, y=w400) -> (x-y=w398:dbl)
              n257 = Subtract(x=w407, y=w406) -> (x-y=w404:dbl)
              n258 = call "move-Motor-v2.vi"("error in"=w394, "Axis"=w405, "Distance (um)"=w404) -> ("error out"=w397:errorcluster)  [unwired: 8 in]
              n259 = call "move-Motor-v2.vi"("error in"=w397, "Axis"=w399, "Distance (um)"=w398) -> ("error out"=w393:errorcluster)  [unwired: 8 in]
            }
            n260 = Multiply(x=w384, y=-1 ("x-1")) -> (x*y=w383:dbl)
            n261 = call "toggleShutter.vi"("Error In"=w379) -> ("error out"=w378:errorcluster)  [unwired: 9 in]
            n262 = call "move-Motor-v2.vi"("error in"=w378, "Axis"=w385, "Distance (um)"=w383) -> ("error out"=w373:errorcluster)  [unwired: 8 in]
          }
          n263 = call "move-Motor-v2.vi"("error in"=w366, "Axis"=w365, "Distance (um)"="scale  z (um)") -> ()  [unwired: 8 in, 1 out]
        }
      }
    }
  }
